vi "PV ActiveLine - DisplayControlContrast.vi"(7 "W/R":bool, 8 "Fehler (Eingang)":errorcluster, 9 "Contrast":u8=40 max=100 step=1, 11 "Referenz in":refnum<visa-resource-name>) -> (0 "Cluster (Ausgang)":errorcluster, 2 "Contrast Out":u8, 3 "Referenz out":refnum<visa-resource-name>)   [LabVIEW 2013, in "PV ActiveLine.lvlib"]
doc: "DCC - Display Control Contrast\n\nTransmit: DCC [,a]\nReceive: a\n\nContrast in percent, a = 0 … 100\n100% = full contrast\ndefault = 40"
uses:
  <instrlib>/PV ActiveLine/PV ActiveLine.lvlib
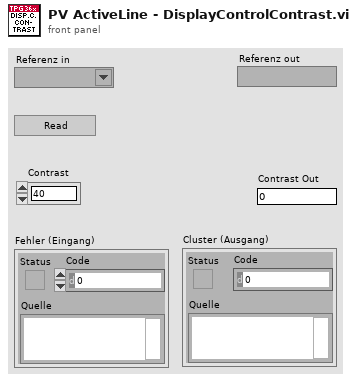
[diagram p1: front panel]
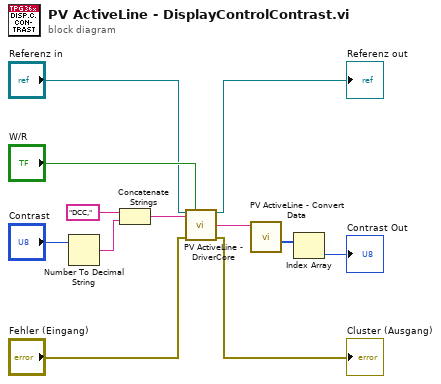
[diagram p0: block diagram]
diagram:
  n1 = Number To Decimal String(number="Contrast") -> (decimal integer string=w8:string)  [unwired: 1 in]
  n2 = Concatenate Strings("DCC,", w8) -> (w10:string)
  n3 = call <instrlib>:"PV ActiveLine - DriverCore.vi"("Referenz in"="Referenz in", "Write/Read"="W/R", "Command"=w10, "Fehler (Eingang)"="Fehler (Eingang)") -> ("Referenz out"=→"Referenz out":refnum<visa-resource-name>, "String Out"=w3:string, "Cluster (Ausgang)"=→"Cluster (Ausgang)":errorcluster)  [unwired: 9 in]
  n4 = call <instrlib>:"PV ActiveLine - Convert Data.vi"("String in"=w3) -> ("Integer Out"=w2:i32[])  [unwired: 7 in, 3 out]
  n5 = Index Array(array=w2) -> (element=→"Contrast Out":i32)  [unwired: 1 in]
